vi "To Center and Span (frequency).vi"(4 "stop":dbl[unit], 6 "start":dbl[unit]) -> (0 "span":dbl[unit], 2 "center":dbl[unit])   [LabVIEW 2017]
doc: "Takes two frequencies that indicate the beginning and end of a frequency range and returns the average (\"center\") and difference (\"span\") of the two frequencies."
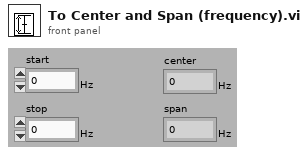
[diagram p1: front panel]
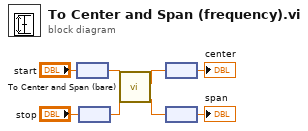
[diagram p0: block diagram]
diagram:
  n1 = node("start") -> (w4:dbl)
  n2 = node("stop") -> (w3:dbl)
  n3 = call "To Center and Span (bare).vi"("stop"=w3, "start"=w4) -> ("span"=w1:dbl, "center"=w2:dbl)  [unwired: 4 out]
  n4 = node(w2) -> (→"center":dbl[unit])
  n5 = node(w1) -> (→"span":dbl[unit])
